vi "Write Setpoint.vi"(8 "error in":errorcluster, 10 "Setpoint":sgl, 11 "Alicat Controller in":refnum<class "Alicat Controller.lvclass">) -> (0 "error out":errorcluster, 2 "SPStr":string, 3 "Alicat Controller out":refnum<class "Alicat Controller.lvclass">)   [LabVIEW 2015, in "Alicat.lvlib" / "Alicat Controller.lvclass"]
doc: "This VI will write the setpoint requested to the private data cluster and translate the setpoint to a string which is understandable to the controller."
uses:
  Alicat Controller.lvclass
  Alicat Controller.lvclass/Alicat Controller.ctl
  Alicat.lvclass
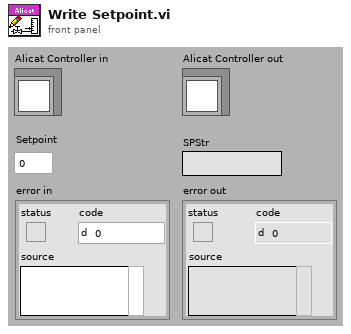
[diagram p1: front panel]
types:
  T1 = typedef "Alicat.lvlib/Alicat.lvclass/CtlSetup.ctl" = cluster{"Name":string, "Address":string, "fullScale":dbl, "Gas":T2}
  T2 = typedef "Alicat.lvlib/Alicat.lvclass/Gas.ctl" = enum16{"Air", "Ar", "CH4", "CO", "CO2", "C2H6", "H2", "He", "N2", "NO", "Ne", "O2", "C3H8", "n-C4H10", "C2H2", "C2H4", "i-C2H10", "Kr", "Xe"}
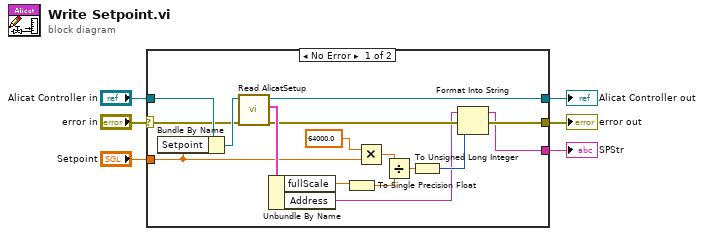
[diagram p0: block diagram]
diagram:
  n1 = case shown="No Error" "error in" {
    selector: "error in" -> [w20 w24]
    tunnel: [w13 w24] -> w5
    tunnel: [w16 w23] -> w3
    tunnel: "Alicat Controller in" -> [w22 w23]
    tunnel: "Setpoint" -> [w15 _]
    tunnel: [w7 _] -> w1
    frame No Error {
      n2 = Bundle By Name(cluster=w22, "Setpoint"=w15) -> (w21:refnum<class "Alicat Controller.lvclass">)
      n3 = call "Read AlicatSetup.vi"("error in (no error)"=w20, "Alicat in"=w21) -> ("error out"=w14:errorcluster, "AlicatSetup"=w17:T1, "Alicat out"=w16:refnum<class "Alicat Controller.lvclass">)  [unwired: 7 in]
      n4 = Unbundle By Name(w17) -> ("fullScale"=w9:dbl, "Address"=w10:string)
      n5 = To Single Precision Float(number=w9) -> (single precision float=w8:sgl)
      n6 = Multiply(x=sgl 64000.0, y=w15) -> (x*y=w18:sgl)
      n7 = Divide(x=w18, y=w8) -> (x/y=w12:sgl)
      n8 = To Unsigned Long Integer(number=w12) -> (unsigned 32bit integer=w11:u32)
      n9 = Format Into String(initial string=w10, error in=w14, w11) -> (resulting string=w7:string, error out=w13:errorcluster)  [unwired: 1 in]
    }
    frame Error {
    }
  }
  "error out" <- w5
  "Alicat Controller out" <- w3
  "SPStr" <- w1
